vi "Port.vi"(8 "error in":errorcluster, 11 "Node Ptr":T1 format="%.0x") -> (0 "error out":errorcluster)   [LabVIEW 2020, in "Ballard MIL-STD-1553 System Explorer.lvlib" / "Implementation.lvlib"]
uses:
  Implementation.lvlib
  <vilib>/NI VeriStand/Custom Device API/Custom Device Item Ref.ctl
  <vilib>/NI VeriStand/Custom Device API/Custom Device API.lvlib
  Scripting/Ballard MIL-STD-1553 Scripting.lvlib
panel:
  out "channel":u16 caption="Channel Number"
  in  "SHDocVw.IWebBrowser":refnum<k7>(container)
  in  "General Header":cluster{"Section Name":string}={"Section Name"="General Page Settings"}
  in  "Description":string
  out "Name":string
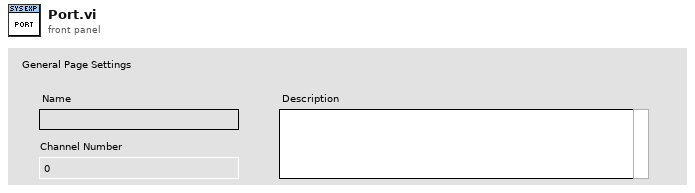
[diagram p1: front panel]
types:
  T1 = typedef "Custom Device API.lvlib/Custom Device Item Ref.ctl" = u64
  T2 = typedef "Custom Device API.lvlib/Custom Device Item Info.ctl" = cluster{"Name":string, "Is Channel":bool, "GUID":string, "Is Waveform":bool}
  T3 = typedef "Custom Device API.lvlib/Custom Device Commands.ctl" = enum16{"Default", "Item renamed", "Shutdown", "Dynamic button pressed"}
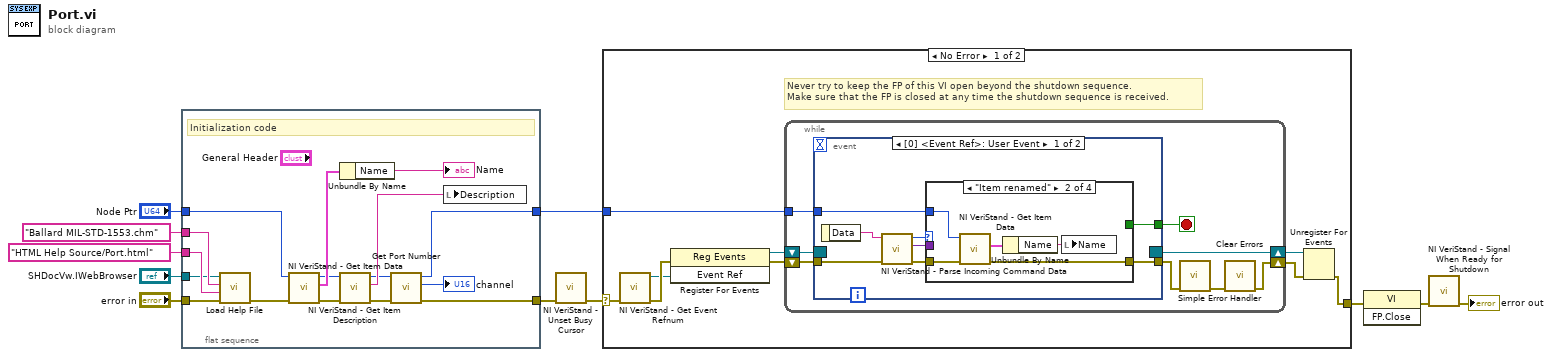
[diagram p0: block diagram]
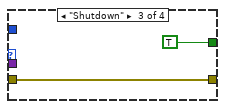
[diagram p3: hidden frame]
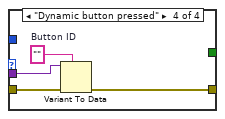
[diagram p4: hidden frame]
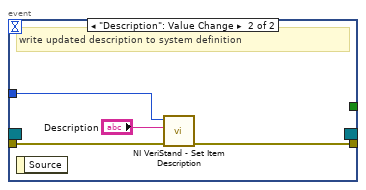
[diagram p5: hidden frame]
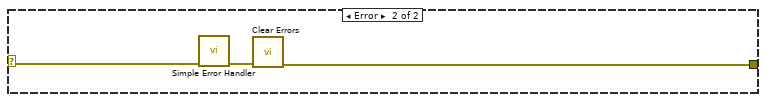
[diagram p6: hidden frame]
diagram:
  n1 = flat-sequence "Initialization code" {
    tunnel: "error in" -> [w25]
    tunnel: "Node Ptr" -> [w17]
    tunnel: [w20] -> w7
    tunnel: [w21] -> w4
    tunnel: "SHDocVw.IWebBrowser" -> [w22]
    tunnel: "HTML Help Source/Port.html" ("CD_CHM_Section") -> [w24]
    tunnel: "Ballard MIL-STD-1553.chm" ("CD_CHM_FileName") -> [w23]
    frame #0 {
      # "Initialization code"
      n2 = call "Load Help File.vi"("error in (no error)"=w25, "HTML File to Load"=w24, "Main CHM File"=w23, "Browser"=w22) -> ("error out"=w18:errorcluster)  [unwired: 7 in]
      n3 = call <vilib>:"NI VeriStand - Get Item Data.vi"("error in (no error)"=w18, "Item Ref in"=w17) -> ("error out"=w15:errorcluster, "Item Info"=w27:T2, "Item Ref out"=w16:T1)  [unwired: 7 out]
      n4 = Unbundle By Name(w27) -> ("Name"=→"Name":string)
      n5 = call <vilib>:"NI VeriStand - Get Item Description.vi"("error in (no error)"=w15, "Item Ref in"=w16) -> ("error out"=w13:errorcluster, "Description"=w26:string, "Item Ref out"=w14:T1)  [unwired: 7 out]
      n6 = call "Get Port Number.vi"("error in"=w13, "port in"=w14) -> ("error out"=w20:errorcluster, "port number"=→"channel":u16, "port out"=w21:T1)  [unwired: 6 in, 1 out]
      n7 = local write "Description"(w26) -> ()
    }
  }
  n8 = call <vilib>:"NI VeriStand - Unset Busy Cursor.vi"("error in (no error)"=w7) -> ("error out"=w6:errorcluster)  [unwired: 10 out]
  n9 = case shown="No Error" w6 {
    selector: w6 -> [w28 w71]
    tunnel: [w33 w69] -> w11
    tunnel: w4 -> [w29 _]
    frame No Error {
      # "Never try to keep the FP of this VI open beyond the shutdown sequence.\nMake sure that the FP is closed at any time the shutdown sequence is received."
      n10 = call <vilib>:"NI VeriStand - Get Event Refnum.vi"("error in (no error)"=w28) -> ("error out"=w36:errorcluster, "Event Ref"=w32:refnum<user-event>)  [unwired: 9 out]
      n11 = register-events(error in=w36, w32) -> (reference out=w30:refnum<event-registration>, error out=w31:errorcluster)  [unwired: 1 in]
      n12 = while {
        tunnel: w29 -> [w40]
        shift-right: [w37] -> w34
        shift-left: w31 -> [w43]
        shift-right: [w44] -> w35
        shift-left: w30 -> [w42]
        stop <- w41 stop-if-true
        n13 = event shown="[0] <Event Ref>: User Event" {
          selector: w42 -> [_ _]
          dyn-events: [_ _] -> w44
          timeout: _ -> [_ _]
          tunnel: w43 -> [w52 w67]
          tunnel: [w49 _] -> w41
          tunnel: [w48 w66] -> w39
          tunnel: w40 -> [w47 w68]
          event User Event {
            n14 = event-data() -> ("Data"=w45:string)  [unwired: 1 out]
            n15 = call <vilib>:"NI VeriStand - Parse Incoming Command Data.vi"("error in (no error)"=w52, "Incoming data"=w45) -> ("error out"=w51:errorcluster, "Outgoing data"=w46:variant, "Action"=w50:T3)  [unwired: 7 out]
            n16 = case shown="\"Item renamed\"" w50 {
              tunnel: w51 -> [w53 w58 w59 w64]
              tunnel: [_ _ TRUE _] -> w49
              tunnel: [w53 w55 w59 w61] -> w48
              tunnel: w47 -> [_ w57 _ _]
              tunnel: w46 -> [_ _ _ w63]
              frame Default {
              }
              frame "Item renamed" {
                n17 = call <vilib>:"NI VeriStand - Get Item Data.vi"("error in (no error)"=w58, "Item Ref in"=w57) -> ("error out"=w55:errorcluster, "Item Info"=w56:T2)  [unwired: 8 out]
                n18 = Unbundle By Name(w56) -> ("Name"=w54:string)
                n19 = local write "Name"(w54) -> ()
              }
              frame "Shutdown" {
              }
              frame "Dynamic button pressed" {
                w62 = ""  # Button ID
                n20 = Variant To Data(error in=w64, type=w62, Variant=w63) -> (error out=w61:errorcluster)  [unwired: 1 out]
              }
            }
          }
          event "Description": Value Change {
            # "write updated description to system definition"
            n21 = event-data() -> ()  [unwired: 2 out]
            n22 = call <vilib>:"NI VeriStand - Set Item Description.vi"("error in (no error)"=w67, "Description"="Description", "Item Ref in"=w68) -> ("error out"=w66:errorcluster)  [unwired: 8 out]
          }
        }
        n23 = call <vilib>:"Simple Error Handler.vi"("error in (no error)"=w39) -> ("error out"=w38:errorcluster)  [unwired: 1 in, 7 out]
        n24 = call <vilib>:"Clear Errors.vi"("error in (no error)"=w38) -> ("error out"=w37:errorcluster)  [unwired: 1 in, 5 out]
      }
      n25 = Unregister For Events(event registration refnum=w35, error in=w34) -> (error out=w33:errorcluster)
    }
    frame Error {
      n26 = call <vilib>:"Simple Error Handler.vi"("error in (no error)"=w71) -> ("error out"=w70:errorcluster)  [unwired: 1 in, 7 out]
      n27 = call <vilib>:"Clear Errors.vi"("error in (no error)"=w70) -> ("error out"=w69:errorcluster)  [unwired: 1 in, 5 out]
    }
  }
  n28 = invoke class="VI" method="FP.Close"(error in=w11) -> (error out=w10:errorcluster)  [unwired: 2 in, 2 out]
  n29 = call <vilib>:"NI VeriStand - Signal When Ready for Shutdown.vi"("error in (no error)"=w10) -> ("error out"=→"error out":errorcluster)  [unwired: 10 out]
